vi "main.vi"   [LabVIEW 2013]
uses:
  030 - EVENTS/EnumFgvEventCommand.ctl
  Class/EVE/EVE_AppSpecific/EVE_AppSpecific.lvclass
  040 - SCREENS/enumScreen.ctl
  090 - ERRORS/Ctrls/enumLogAndView.ctl
  <vilib>/Utility/error.llb/DialogType.ctl
  Class/EVE/EVE.lvclass
panel:
  # "MAIN"
types:
  T1 = typedef "EnumFgvEventCommand.ctl" = enum16{"Setup", "Cleanup", "Get"}
  T2 = enum32{"Invalid", "Standard", "Closed", "Hidden", "Minimized", "Maximized"}
  T3 = typedef "enumLogAndView.ctl" = enum16{"Log only", "Log and view"}
  T4 = typedef "enumScreen.ctl" = enum16{"Test screen", "Ecran principal", "LOG", "Setup", "Popup : About", "Popup : View last message", "Popup : WebBrowser help", "Traduction", "Popup : DEBUG Process"}
  T5 = typedef "DialogType.ctl" = u16
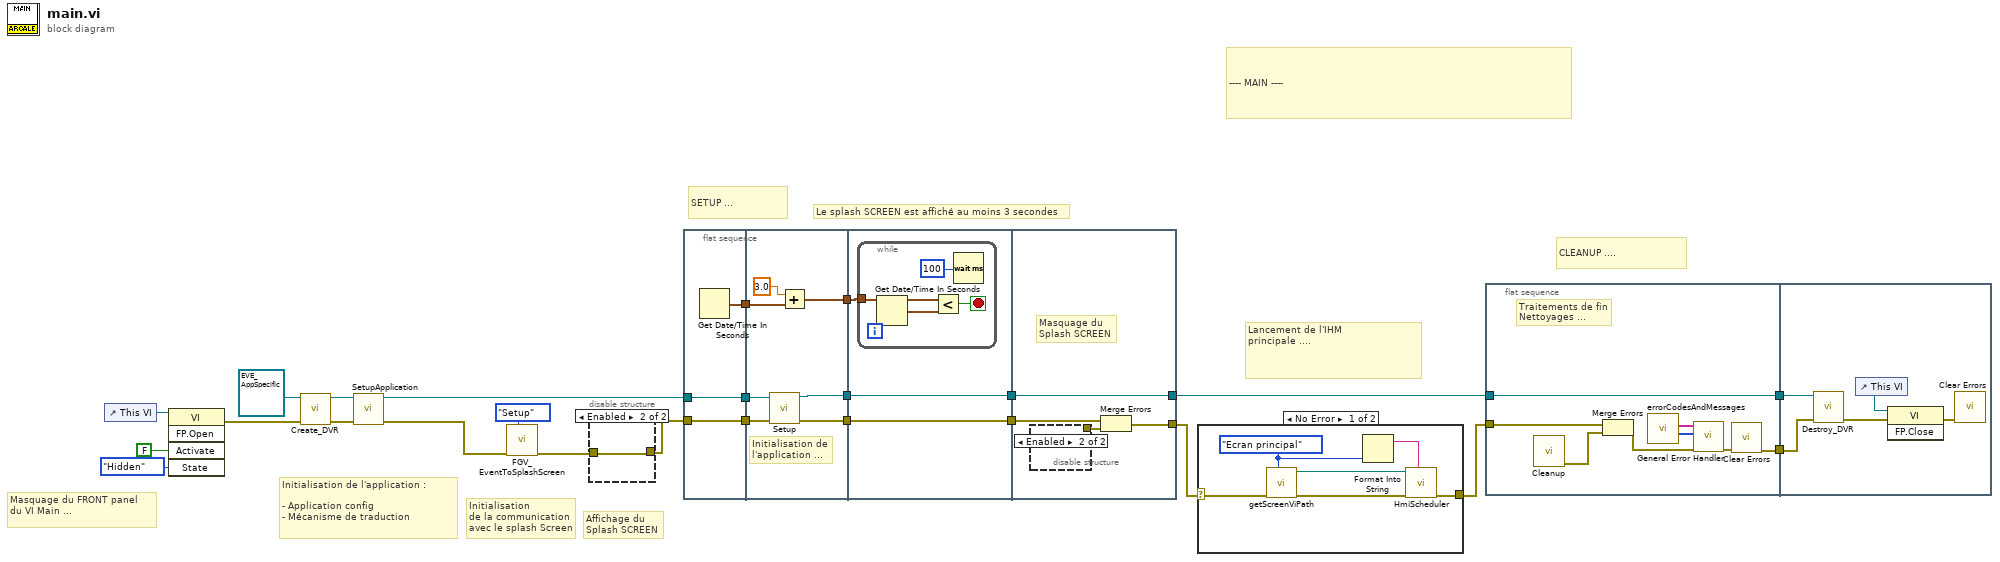
[diagram p0: block diagram]
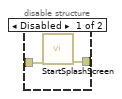
[diagram p2: hidden frame]
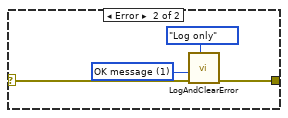
[diagram p3: hidden frame]
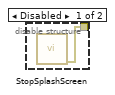
[diagram p4: hidden frame]
diagram:
  # "Initialisation de l'application :\n\n- Application config\n- Mécanisme de traduction"
  # "CLEANUP ...."
  # "SETUP ..."
  # "Le splash SCREEN est affiché au moins 3 secondes"
  # "Lancement de l'IHM\nprincipale ...."
  # "Initialisation\nde la communication\navec le splash Screen"
  # "Masquage du FRONT panel\ndu VI Main ..."
  # "Affichage du\nSplash SCREEN"
  # "---- MAIN ----"
  n1 = control-ref of="This VI"() -> (w25:refnum<vi>)
  n2 = invoke class="VI" method="FP.Open"(reference=w25, "Activate"=FALSE ("Activate?"), "State"=T2."Hidden") -> (error out=w10:errorcluster)  [unwired: 2 in, 4 out]
  n3 = call-dynamic "Create_DVR.vi"("error in (no error)"=w10, "EVE in"=refnum<class "EVE_AppSpecific.lvclass"> refnum ("EVE_AppSpecific.lvclass")) -> ("error out"=w9:errorcluster, "EVE reference"=w3:refnum<data-value>)  [unwired: 8 in]
  n4 = call "SetupApplication.vi"("error in (no error)"=w9, "EVE reference in"=w3) -> ("error out"=w14:errorcluster, "EVE reference out"=w2:refnum<data-value>)  [unwired: 8 in]
  n5 = call "FGV_EventToSplashScreen.vi"("Command"=EnumFgvEventCommand."Setup", "error in (no error)"=w14) -> ("error out"=w13:errorcluster)  [unwired: 8 in, 1 out]
  n6 = disable-structure shown="Enabled" {
    disable-tunnel: w13 -> [w27 w28]
    disable-tunnel: [w26 w28] -> w12
    frame Disabled {
      n7 = call "StartSplashScreen.vi"("error in (no error)"=w27) -> ("error out"=w26:errorcluster)  [unwired: 10 in]
    }
    frame Enabled {
    }
  }
  n8 = flat-sequence {
    tunnel: w12 -> [w31]
    tunnel: [w31] -> w21
    tunnel: [w30] -> w20
    tunnel: w2 -> [w29]
    tunnel: [w29] -> w8
    tunnel: w21 -> [w38]
    tunnel: w20 -> [w37]
    tunnel: [w35] -> w19
    tunnel: [w34] -> w11
    tunnel: w8 -> [w33]
    tunnel: [w32] -> w7
    tunnel: w19 -> [w41]
    tunnel: [w40] -> w17
    tunnel: w11 -> [w40]
    tunnel: w7 -> [w39]
    tunnel: [w39] -> w6
    tunnel: [w48] -> w15
    tunnel: w17 -> [w49]
    tunnel: [w46] -> w5
    tunnel: w6 -> [w46]
    frame #0 {
      n9 = Get Date/Time In Seconds() -> (seconds since 1Jan1904=w30:timestamp)
    }
    frame #1 {
      # "Initialisation de\nl'application ..."
      n10 = call "Setup.vi"("Error in"=w38, "EVE reference in"=w33) -> ("error out"=w34:errorcluster, "EVE reference out"=w32:refnum<data-value>)  [unwired: 8 in]
      n11 = Add(x=3.0, y=w37) -> (x+y=w35:timestamp)
    }
    frame #2 {
      n12 = while {
        tunnel: w41 -> [w43]
        stop <- w45 stop-if-true
        n13 = Get Date/Time In Seconds() -> (seconds since 1Jan1904=w44:timestamp)
        n14 = Less?(x=w43, y=w44) -> (x < y?=w45:bool)
        n15 = Wait (ms)(milliseconds to wait=u32 100) -> ()  [unwired: 1 out]
      }
    }
    frame #3 {
      # "Masquage du\nSplash SCREEN"
      n16 = disable-structure shown="Enabled" {
        disable-tunnel: [w50 _] -> w47
        frame Disabled {
          n17 = call "StopSplashScreen.vi"() -> ("error out"=w50:errorcluster)  [unwired: 11 in]
        }
        frame Enabled {
        }
      }
      n18 = Merge Errors(w49, w47) -> (w48:errorcluster)
    }
  }
  n19 = case shown="No Error" w15 {
    selector: w15 -> [w51 w59]
    tunnel: [w52 w60] -> w18
    frame No Error {
      w54 = enumScreen."Ecran principal" ("Enum Screen")
      n20 = call "getScreenViPath.vi"("Enum Screen"=w54, "error in (no error)"=w51) -> ("error out"=w56:errorcluster, "Path"=w55:path)  [unwired: 8 in]
      n21 = Format Into String(w54) -> (resulting string=w53:string)  [unwired: 3 in, 1 out]
      n22 = call "HmiScheduler.vi"("Param Screen Title"=w53, "error in (no error)"=w56, "Param Initial VI Path"=w55) -> ("error out"=w52:errorcluster)  [unwired: 8 in]
    }
    frame Error {
      w57 = T5 1 items=["no dialog", "OK message", "continue or stop message", "OK message + warnings", "continue/stop + warnings"] ("type of dialog")
      n23 = call "LogAndClearError.vi"("Log and view ?"=enumLogAndView."Log only", "error in (no error)"=w59, "type of dialog"=w57) -> ("error out"=w60:errorcluster)  [unwired: 8 in]
    }
  }
  n24 = flat-sequence {
    tunnel: [w62] -> w16
    tunnel: w18 -> [w68]
    tunnel: w5 -> [w61]
    tunnel: [w61] -> w4
    tunnel: w16 -> [w71]
    tunnel: w4 -> [w69]
    frame #0 {
      # "Traitements de fin\nNettoyages ..."
      n25 = call "Cleanup.vi"() -> ("error out"=w67:errorcluster)  [unwired: 11 in]
      n26 = Merge Errors(w68, w67) -> (w66:errorcluster)
      n27 = call "errorCodesAndMessages.vi"() -> ("errorCodes"=w64:i32[], "errorMessages"=w65:string[])  [unwired: 10 in]
      n28 = call <vilib>:"General Error Handler.vi"("[user-defined codes]"=w64, "[user-defined descriptions]"=w65, "error in (no error)"=w66) -> ("error out"=w63:errorcluster)  [unwired: 8 in, 4 out]
      n29 = call <vilib>:"Clear Errors.vi"("error in (no error)"=w63) -> ("error out"=w62:errorcluster)  [unwired: 6 in]
    }
    frame #1 {
      n30 = call "Destroy_DVR.vi"("error in (no error)"=w71, "EVE reference"=w69) -> ("error out"=w70:errorcluster)  [unwired: 8 in, 1 out]
      n31 = control-ref of="This VI"() -> (w73:refnum<vi>)
      n32 = invoke class="VI" method="FP.Close"(reference=w73, error in=w70) -> (error out=w72:errorcluster)  [unwired: 1 in, 2 out]
      n33 = call <vilib>:"Clear Errors.vi"("error in (no error)"=w72) -> ()  [unwired: 6 in, 1 out]
    }
  }
